vi "jv_keithley-2400.vi"(5 "Cell details cluster":T1, 6 "intensity (no. of suns)":string, 7 "Scan settings":T2 {"J-t settling delay (s)" min=0.0; "J-t illumination" items=["Light only", "Dark only", "Light then dark", "Dark then light"]; "Measurement speed" items=["Fast", "Normal", "High accuracy"]; "Illumination" items=["Light only", "Dark only", "Light then dark", "Dark then light"]; "Only repeat for best pixel" items=["only for best pixel", "for best 2 pixels", "for best 3 pixels", "for best 4 pixels", "for best 5 pixels", "for best 6 pixels", "for best 7 pixels", "for all pixels"]; "No. of repeat scans" min=1.0 step=1.0; "Max power best pixel only" items=["only the best pixel", "the best 2 pixels", "the best 3 pixels", "the best 4 pixels", "the best 5 pixels", "the best 6 pixels", "the best 7 pixels", "all pixels"]; "J-t best pixel only" items=["only the best pixel", "the best 2 pixels", "the best 3 pixels", "the best 4 pixels", "the best 5 pixels", "the best 6 pixels", "the best 7 pixels", "all pixels"]; "J-t measurement speed" items=["Fast", "Normal", "High Accuracy"]; "Stabilisation mode" items=["V", "I"]; "Measurement delay (ms)" min=10.0}, 10 "File path for jv data":path, 11 "VISA Refnum in":refnum<visa-resource-name>) -> (0 "error out":errorcluster, 1 "1st scan direction":string, 2 "HL jv metrics":string[](array[string]), 3 "LH jv metrics":string[](array[string]))   [LabVIEW 2016]
uses:
  TypeDefs/scan_settings.ctl
  <instrlib>/Keithley 24XX/Public/Data/Read (Single Point).vi
  <instrlib>/Keithley 24XX/Keithley 24XX.lvlib
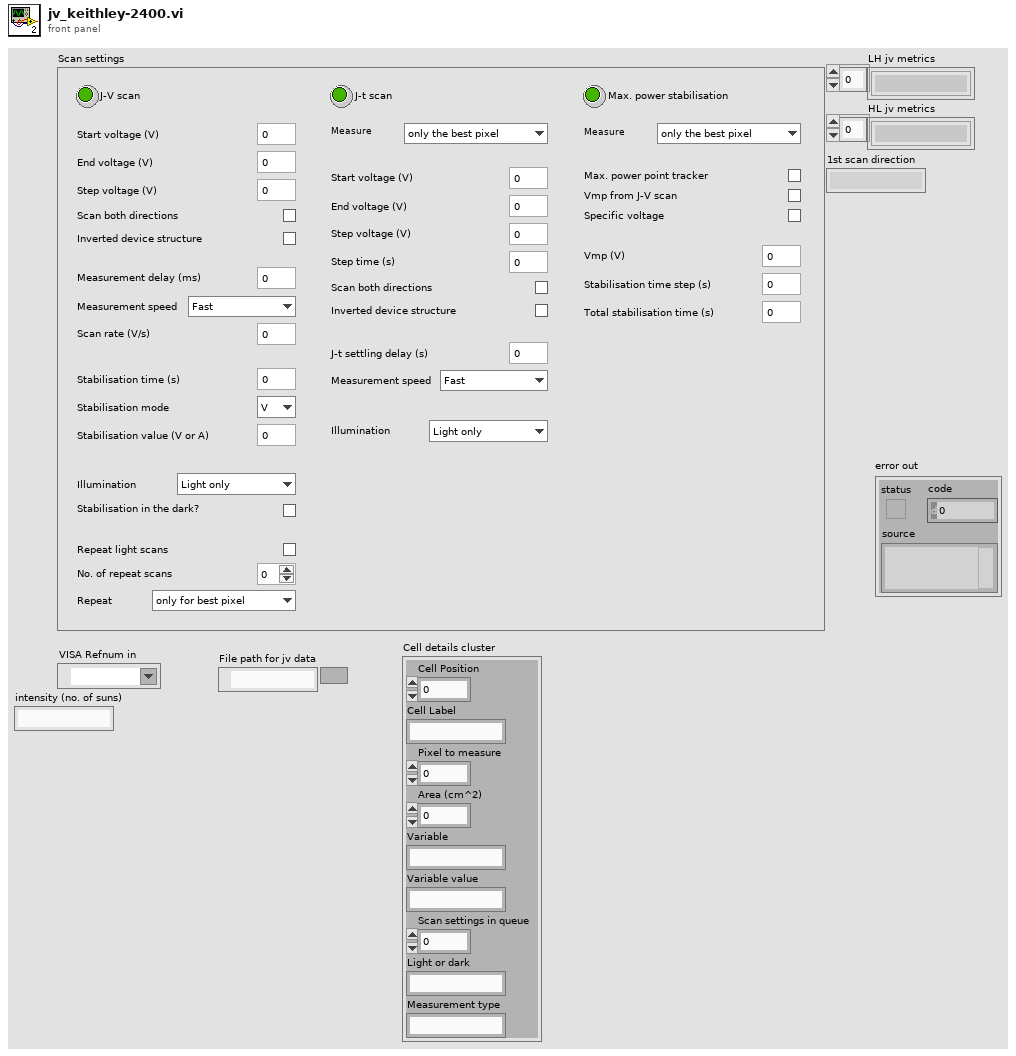
[diagram p1: front panel]
types:
  T1 = cluster{"Cell Position":i32, "Cell Label":string, "Pixel to measure":u16, "Area (cm^2)":dbl, "Variable":string, "Variable value":string, "Scan settings in queue":u16, "Light or dark":string, "Measurement type":string}
  T2 = typedef "scan_settings.ctl" = cluster{"J-V scan":bool, "Start voltage (V)":dbl, "End voltage (V)":dbl, "Step voltage (V)":dbl, "Scan both directions":bool, "Inverted device structure":bool, "Measurement delay (ms)":dbl, "Measurement speed":u8, "Scan rate (V/s)":dbl, "Stabilisation time (s)":dbl, "Stabilisation mode":u16, "Stabilisation value (V or A) ":dbl, "Illumination":u16, "Stabilisation in the dark?":bool, "Repeat light scans":bool, "No. of repeat scans":dbl, "Only repeat for best pixel":u16, "J-t scan":bool, "J-t best pixel only":u16, "J-t start voltage (V)":dbl, "J-t end voltage (V)":dbl, "J-t step voltage (V)":dbl, "Step time (s)":dbl, "J-t scan both directions":bool, "J-t inverted device structure":bool, "J-t settling delay (s)":dbl, "J-t measurement speed":u16, "J-t illumination":u16, "Max. power stabilisation":bool, "Max power best pixel only":u16, "Max. power point tracker":bool, "Vmp from J-V scan":bool, "Max P stab. Specific voltage":bool, "Vmp (V)":dbl, "Stabilisation time step (s)":dbl, "Total stabilisation time (s)":dbl}
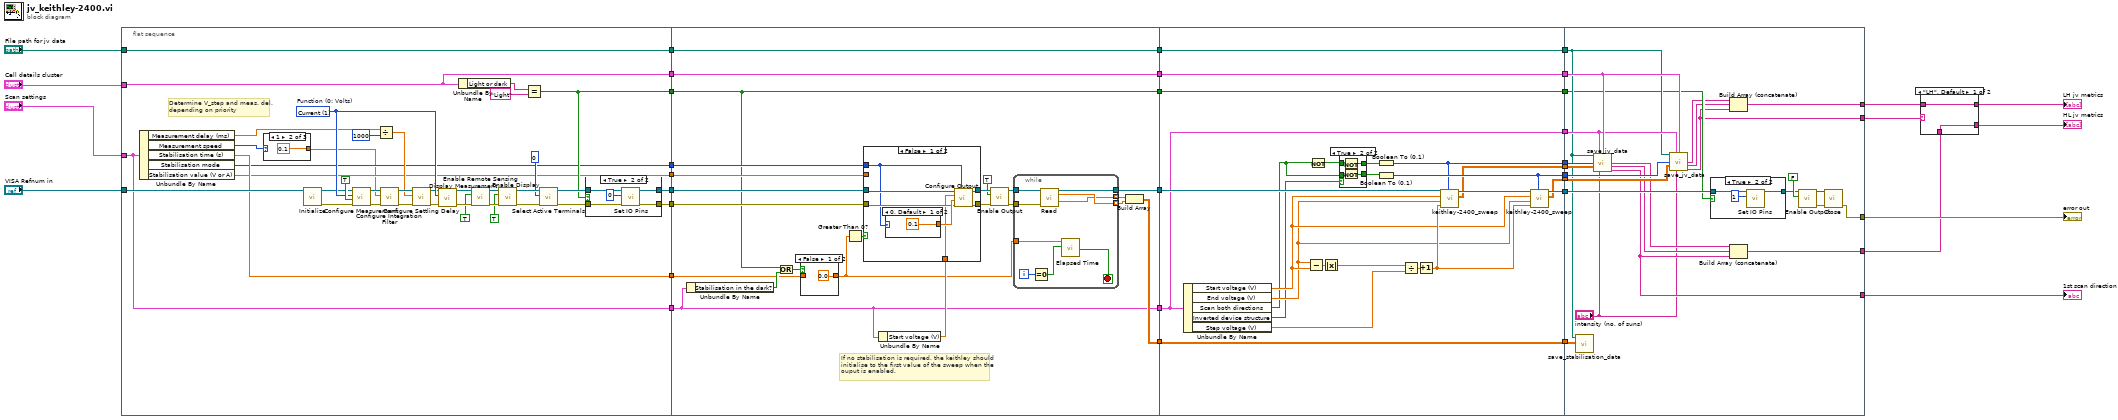
[diagram p0: block diagram]
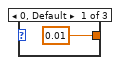
[diagram p3: hidden frame]
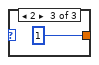
[diagram p4: hidden frame]
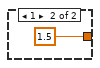
[diagram p7: hidden frame]
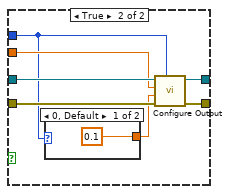
[diagram p8: hidden frame]
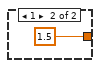
[diagram p9: hidden frame]
diagram:
  n1 = flat-sequence {
    tunnel: [w41] -> w36
    tunnel: [w55] -> w35
    tunnel: [w56] -> w34
    tunnel: [w40] -> w33
    tunnel: [w42] -> w32
    tunnel: [w37] -> w31
    tunnel: [w45] -> w30
    tunnel: [w48] -> w29
    tunnel: [w46] -> w28
    tunnel: "File path for jv data" -> [w46]
    tunnel: "Cell details cluster" -> [w45]
    tunnel: "VISA Refnum in" -> [w44]
    tunnel: "Scan settings" -> [w37]
    tunnel: w36 -> [w96]
    tunnel: w35 -> [w104]
    tunnel: w34 -> [w105]
    tunnel: [w100] -> w27
    tunnel: [w97] -> w26
    tunnel: w33 -> [w94]
    tunnel: w32 -> [w87]
    tunnel: [w91] -> w25
    tunnel: w31 -> [w91]
    tunnel: [w95] -> w24
    tunnel: w30 -> [w95]
    tunnel: w29 -> [w85]
    tunnel: w28 -> [w86]
    tunnel: [w86] -> w23
    tunnel: [w85] -> w7
    tunnel: [w156] -> w22
    tunnel: w27 -> [w160]
    tunnel: w26 -> [w145]
    tunnel: w25 -> [w138]
    tunnel: w24 -> [w139]
    tunnel: w23 -> [w140]
    tunnel: [w145] -> w16
    tunnel: [w144] -> w15
    tunnel: [w143] -> w14
    tunnel: [w142] -> w13
    tunnel: [w141] -> w12
    tunnel: [w140] -> w11
    tunnel: [w139] -> w10
    tunnel: [w138] -> w9
    tunnel: [w137] -> w8
    tunnel: w7 -> [w137]
    tunnel: w22 -> [w187]
    tunnel: [w185] -> w17
    tunnel: w16 -> [w184]
    tunnel: w15 -> [w183]
    tunnel: w14 -> [w182]
    tunnel: w13 -> [w181]
    tunnel: w12 -> [w180]
    tunnel: w11 -> [w177]
    tunnel: w10 -> [w179]
    tunnel: w9 -> [w178]
    tunnel: w8 -> [w176]
    tunnel: [w171] -> w6
    tunnel: [w170] -> w5
    tunnel: [w169] -> w3
    tunnel: [w168] -> w1
    frame #0 {
      w71 = u16 1 items=["Volts", "Current", "Resistance"]  # Function (0: Volts)
      # "Determine V_step and meas. del.\ndepending on priority"
      n2 = Unbundle By Name(w37) -> ("Measurement delay (ms)"=w38:dbl, "Measurement speed"=w43:u8, "Stabilisation time (s)"=w42:dbl, "Stabilisation mode"=w40:u16, "Stabilisation value (V or A)"=w41:dbl)
      n3 = case shown="1" w43 {
        tunnel: [0.01 0.1 1] -> w39
        frame 0, Default {
        }
        frame 1 {
        }
        frame 2 {
        }
      }
      n4 = call <instrlib>:"Initialize.vi"("VISA resource name"=w44) -> ("error out"=w61:errorcluster, "VISA resource name out"=w62:refnum<visa-resource-name>)  [unwired: 4 in, 5 out]
      n5 = call <instrlib>:"Configure Measurement.vi"("error in (no error)"=w61, "Enable Auto Range (T:Enable)"=TRUE, "Function (0: Volts)"=w71, "VISA resource name"=w62) -> ("error out"=w64:errorcluster, "VISA resource name out"=w63:refnum<visa-resource-name>)  [unwired: 6 in]
      n6 = Divide(x=w38, y=1000) -> (x/y=w70:dbl)
      n7 = call <instrlib>:"Configure Integration Filter.vi"("error in (no error)"=w64, "Measurement Speed (1 PLC)"=w39, "VISA resource name"=w63) -> ("error out"=w73:errorcluster, "VISA resource name out"=w72:refnum<visa-resource-name>)  [unwired: 7 in]
      n8 = call <instrlib>:"Configure Settling Delay.vi"("error in (no error)"=w73, "Manual Settling Delay (0 sec)"=w70, "VISA resource name"=w72) -> ("error out"=w68:errorcluster, "VISA resource name out"=w67:refnum<visa-resource-name>)  [unwired: 7 in]
      n9 = call <instrlib>:"Display Measurement.vi"("error in (no error)"=w68, "Displayed Measurement (0: Voltage)"=w71, "VISA resource name"=w67) -> ("error out"=w66:errorcluster, "VISA resource name out"=w65:refnum<visa-resource-name>)  [unwired: 7 in]
      n10 = Unbundle By Name(w45) -> ("Light or dark"=w54:string)
      n11 = call <instrlib>:"Enable Remote Sensing.vi"("error in (no error)"=w66, "Enable Remote Sensing (T: Enable)"=TRUE ("Enable Output (T: Enable)"), "VISA resource name"=w65) -> ("error out"=w59:errorcluster, "VISA resource name out"=w60:refnum<visa-resource-name>)  [unwired: 7 in]
      n12 = call <instrlib>:"Enable Display.vi"("error in (no error)"=w59, "Enable Display (T: Enable)"=TRUE, "VISA resource name"=w60) -> ("error out"=w52:errorcluster, "VISA resource name out"=w53:refnum<visa-resource-name>)  [unwired: 7 in]
      n13 = Equal?(x=w54, y="Light") -> (x = y?=w48:bool)
      n14 = call <instrlib>:"Select Active Terminals.vi"("error in (no error)"=w52, "Active Terminals (0: Front)"=0, "VISA resource name"=w53) -> ("error out"=w50:errorcluster, "VISA resource name out"=w51:refnum<visa-resource-name>)  [unwired: 7 in]
      n15 = case shown="True" w48 {
        tunnel: w51 -> [w79 w83]
        tunnel: w50 -> [w78 w82]
        tunnel: [w79 w81] -> w56
        tunnel: [w78 w80] -> w55
        frame False {
        }
        frame True {
          n16 = call <instrlib>:"Set IO Pins.vi"("error in (no error)"=w82, "Output Pattern (0)"=0, "VISA resource name"=w83) -> ("error out"=w80:errorcluster, "VISA resource name out"=w81:refnum<visa-resource-name>)  [unwired: 7 in]
        }
      }
    }
    frame #1 {
      # "If no stabilisation is required, the keithley should\ninitialise to the first value of the sweep when the\nouput is enabled."
      n17 = Unbundle By Name(w91) -> ("Stabilisation in the dark?"=w90:bool)
      n18 = Or(x=w85, y=w90) -> (x .or. y?=w89:bool)
      n19 = case shown="False" w89 {
        tunnel: [0.0 ("Stabilisation time (s)") w109] -> w88
        tunnel: w87 -> [_ w109]
        frame False {
        }
        frame True {
        }
      }
      n20 = Greater Than 0?(x=w88) -> (x > 0?=w93:bool)
      n21 = Unbundle By Name(w91) -> ("Start voltage (V)"=w92:dbl)
      n22 = case shown="False" w93 {
        tunnel: [w114 w125] -> w107
        tunnel: [w115 w124] -> w106
        tunnel: w105 -> [w112 w123]
        tunnel: w104 -> [w113 w122]
        tunnel: w96 -> [_ w121]
        tunnel: w94 -> [w111 w120]
        tunnel: w92 -> [w110 _]
        frame False {
          n23 = case shown="0, Default" w111 {
            tunnel: [0.1 1.5] -> w116
            frame 0, Default {
            }
            frame 1 {
            }
          }
          n24 = call <instrlib>:"Configure Output.vi"("Source Mode  (0: Voltage)"=w111, "error in (no error)"=w113, "Compliance  Level (0.1)"=w116, "Output Level (0)"=w110, "VISA resource name"=w112) -> ("error out"=w114:errorcluster, "VISA resource name out"=w115:refnum<visa-resource-name>)  [unwired: 5 in]
        }
        frame True {
          n25 = case shown="0, Default" w120 {
            tunnel: [0.1 1.5] -> w119
            frame 0, Default {
            }
            frame 1 {
            }
          }
          n26 = call <instrlib>:"Configure Output.vi"("Source Mode  (0: Voltage)"=w120, "error in (no error)"=w122, "Compliance  Level (0.1)"=w119, "Output Level (0)"=w121, "VISA resource name"=w123) -> ("error out"=w125:errorcluster, "VISA resource name out"=w124:refnum<visa-resource-name>)  [unwired: 5 in]
        }
      }
      n27 = call <instrlib>:"Enable Output.vi"("error in (no error)"=w107, "Enable Output (T: Enable)"=TRUE ("Output (Off)"), "VISA resource name"=w106) -> ("error out"=w101:errorcluster, "VISA resource name out"=w102:refnum<visa-resource-name>)  [unwired: 7 in]
      n28 = while {
        tunnel: w102 -> [w136]
        tunnel: w101 -> [w135]
        tunnel: [w134] -> w100
        tunnel: [w128] -> w99 mode=indexing
        tunnel: [w132] -> w98 mode=indexing
        tunnel: w88 -> [w129]
        i -> [w131]
        stop <- w133 stop-if-true
        n29 = Equal To 0?(x=w131) -> (x = 0?=w130:bool)
        n30 = call-poly <instrlib>:"Read.vi"("VISA resource name"=w136, "error in (no error)"=w135) -> ("VISA resource name out"=w134:refnum<visa-resource-name>, "Current"=w132:sgl, "Timestamp"=w128:sgl)  [unwired: 7 in, 4 out]
        n31 = call "Elapsed Time"("Time Target (s)"=w129, "Reset"=w130) -> ("Time has Elapsed"=w133:bool)  [unwired: 10 in, 7 out]
      }
      n32 = Build Array(w99, w98) -> (w97:sgl[][])
    }
    frame #2 {
      n33 = Unbundle By Name(w138) -> ("Start voltage (V)"=w151:dbl, "End voltage (V)"=w150:dbl, "Scan both directions"=w147:bool, "Inverted device structure"=w149:bool, "Step voltage (V)"=w146:dbl)
      n34 = Subtract(x=w150, y=w151) -> (x-y=w158:dbl)
      n35 = Not(x=w147) -> (.not. x?=w148:bool)
      n36 = Absolute Value(x=w158) -> (abs(x)=w159:dbl)
      n37 = case shown="True" w149 {
        tunnel: [w162 w166] -> w153
        tunnel: [w161 w165] -> w152
        tunnel: w147 -> [w161 w164]
        tunnel: w148 -> [w162 w163]
        frame False {
        }
        frame True {
          n38 = Not(x=w163) -> (.not. x?=w166:bool)
          n39 = Not(x=w164) -> (.not. x?=w165:bool)
        }
      }
      n40 = Boolean To (0,1)(Boolean=w153) -> (0, 1=w142:i16)
      n41 = Boolean To (0,1)(Boolean=w152) -> (0, 1=w143:i16)
      n42 = Divide(x=w159, y=w146) -> (x/y=w155:dbl)
      n43 = Increment(x=w155) -> (x+1=w154:dbl)
      n44 = call "keithley-2400_sweep.vi"("Sweep Direction"=w142, "Number of Points"=w154, "Maximum Amplitude"=w150, "Minimum Amplitude"=w151, "VISA resource name out 2"=w160) -> ("Data Array"=w141:dbl[][], "VISA resource name out"=w157:refnum<visa-resource-name>)  [unwired: 2 in, 1 out]
      n45 = call "keithley-2400_sweep.vi"("Sweep Direction"=w143, "Number of Points"=w154, "Maximum Amplitude"=w150, "Minimum Amplitude"=w151, "VISA resource name out 2"=w157) -> ("Data Array"=w144:dbl[][], "VISA resource name out"=w156:refnum<visa-resource-name>)  [unwired: 2 in, 1 out]
    }
    frame #3 {
      n46 = call "save_stabilisation_data.vi"("Stabilisation Data"=w184, "File path for jv data (without scan direction)"=w177) -> ()  [unwired: 10 in]
      n47 = call "save_jv_data.vi"("File path for jv data (without scan direction)"=w177, "Scan settings"=w178, "Cell details cluster"=w179, "Scan direction"=w181, "Data Array"=w180, "intensity (no. of suns)"="intensity (no. of suns)") -> ("j-v metrics"=w173:string[], "File path out (with scan direction)"=w172:string, "scan direction"=w168:string)  [unwired: 5 in, 2 out]
      n48 = call "save_jv_data.vi"("File path for jv data (without scan direction)"=w177, "Scan settings"=w178, "Cell details cluster"=w179, "Scan direction"=w182, "Data Array"=w183, "intensity (no. of suns)"="intensity (no. of suns)") -> ("j-v metrics"=w175:string[], "File path out (with scan direction)"=w174:string, "scan direction"=w171:string)  [unwired: 5 in, 2 out]
      n49 = case shown="True" w176 {
        tunnel: w187 -> [w191 w193]
        tunnel: [w191 w192] -> w186
        frame False {
        }
        frame True {
          n50 = call <instrlib>:"Set IO Pins.vi"("Output Pattern (0)"=1, "VISA resource name"=w193) -> ("VISA resource name out"=w192:refnum<visa-resource-name>)  [unwired: 8 in, 1 out]
        }
      }
      n51 = Build Array (concatenate)(w175, w174, w171) -> (w170:string[])
      n52 = Build Array (concatenate)(w173, w172, w168) -> (w169:string[])
      n53 = call <instrlib>:"Enable Output.vi"("Enable Output (T: Enable)"=FALSE ("Output (Off)"), "VISA resource name"=w186) -> ("error out"=w189:errorcluster, "VISA resource name out"=w190:refnum<visa-resource-name>)  [unwired: 8 in]
      n54 = call <instrlib>:"Close.vi"("error in (no error)"=w189, "VISA resource name"=w190) -> ("error out"=w185:errorcluster)  [unwired: 9 in]
    }
  }
  n55 = case shown="\"LH\", Default" w6 {
    tunnel: w5 -> [w196 w198]
    tunnel: [w196 w197] -> w4
    tunnel: w3 -> [w195 w197]
    tunnel: [w195 w198] -> w2
    frame "LH", Default {
    }
    frame "HL" {
    }
  }
  "LH jv metrics" <- w4
  "HL jv metrics" <- w2
  "error out" <- w17
  "1st scan direction" <- w1
